vi "Pickering 4 Wire Asynchronous.vi"(8 "error in (no error)":errorcluster, 9 "Y Channel Array":string[][](array[string]), 10 "X Channel Array":string[](array[string]), 11 "Control Experiment in":refnum<class "Control Experiment.lvclass">) -> (0 "error out":errorcluster, 3 "Control Experiment out":refnum<class "Control Experiment.lvclass">)   [LabVIEW 2020, in "Control Experiment.lvclass"]
uses:
  Control Experiment.lvclass
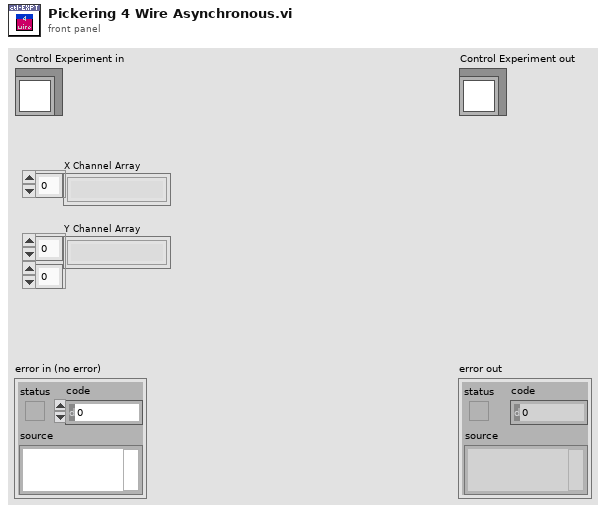
[diagram p1: front panel]
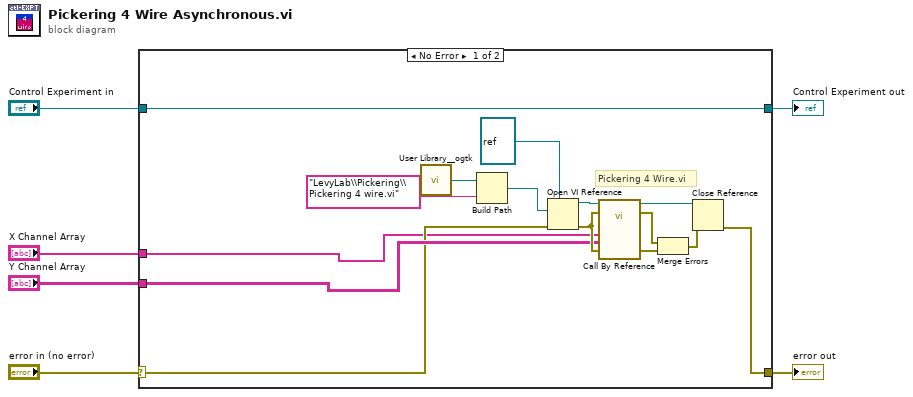
[diagram p0: block diagram]
diagram:
  n1 = case shown="No Error" "error in (no error)" {
    selector: "error in (no error)" -> [w9 w23]
    tunnel: [w8 w23] -> w5
    tunnel: [w21 w22] -> w3
    tunnel: "Control Experiment in" -> [w21 w22]
    tunnel: "Y Channel Array" -> [w10 _]
    tunnel: "X Channel Array" -> [w7 _]
    frame No Error {
      # "Pickering 4 Wire.vi"
      n2 = call <userlib>:"User Library__ogtk.vi"() -> ("User Library (+ Relative)"=w14:path)  [unwired: 1 in]
      n3 = Build Path(base path=w14, name or relative path="LevyLab\\Pickering\\Pickering 4 wire.vi") -> (appended path=w11:path)
      n4 = Open VI Reference(type specifier VI Refnum (for type only)=refnum<vi> refnum, vi path=w11, error in (no error)=w9) -> (vi reference=w20:refnum<vi>, error out=w13:errorcluster)  [unwired: 3 in]
      n5 = call-by-ref "?"(reference=w20, error in=w13, 8:"error in (no error)"=w13, "Y Channels"=w10, "X Channels"=w7) -> (reference out=w18:refnum<vi>, error out=w17:errorcluster, 0:"error out"=w16:errorcluster)  [unwired: 7 in, 1 out]
      n6 = Merge Errors(w17, w16) -> (w15:errorcluster)
      n7 = Close Reference(reference=w18, error in (no error)=w15) -> (error out=w8:errorcluster)
    }
    frame Error {
    }
  }
  "error out" <- w5
  "Control Experiment out" <- w3
